vi "Main.vi"(8 "error in":errorcluster, 11 "TCP Listener in":refnum<class "DS TCP Listener.lvclass">) -> (0 "error out":errorcluster, 3 "TCP Listener out":refnum<class "DS TCP Listener.lvclass">)   [LabVIEW 2017, in "DS TCP Server.lvlib" / "DS TCP Listener.lvclass"]
doc: "The <b>Queued Message Handler</b> of the Worker that owns this VI."
uses:
  DS TCP Listener.lvclass
  Initialization Data.ctl
  Response Cases.ctl
  <vilib>/addons/_Workers/Library/Case Label.ctl
  DS TCP Listener.lvclass/DS TCP Listener.ctl
  rqp_Listen for Connections.ctl
  rsp_Add Listener.ctl
  rsp_New Connection.ctl
  <vilib>/addons/_Workers/Library/Classes/Message/Priority.ctl
  <vilib>/addons/_Workers/Library/Workers.lvlib
  <vilib>/addons/_Workers/Library/Classes/Message/Message.lvclass
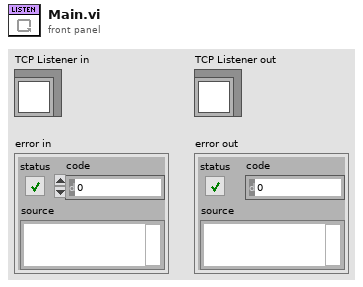
[diagram p1: front panel]
types:
  T1 = typedef "DS TCP Server.lvlib/DS TCP Listener.lvclass/Initialization Data.ctl" = cluster{"Response Cases":T2}
  T2 = typedef "DS TCP Server.lvlib/DS TCP Listener.lvclass/Response Cases.ctl" = cluster{"Add Listener":T3, "New Connection":T3}
  T3 = typedef "Workers.lvlib/Case Label.ctl" = string
  T4 = typedef "DS TCP Server.lvlib/DS TCP Listener.lvclass/rsp_Add Listener.ctl" = cluster{"listener ID":refnum<k5>, "Port":u16}
  T5 = typedef "DS TCP Server.lvlib/DS TCP Listener.lvclass/rqp_Listen for Connections.ctl" = cluster{"Server Name":string, "Port":u16}
  T6 = typedef "DS TCP Server.lvlib/DS TCP Listener.lvclass/rsp_New Connection.ctl" = cluster{"Connection Ref":refnum<k5>, "Name":string, "Message Priority":T7, "IP Address":string}
  T7 = typedef "Workers.lvlib/Message.lvclass/Priority.ctl" = enum16{"Low", "Normal", "High"}
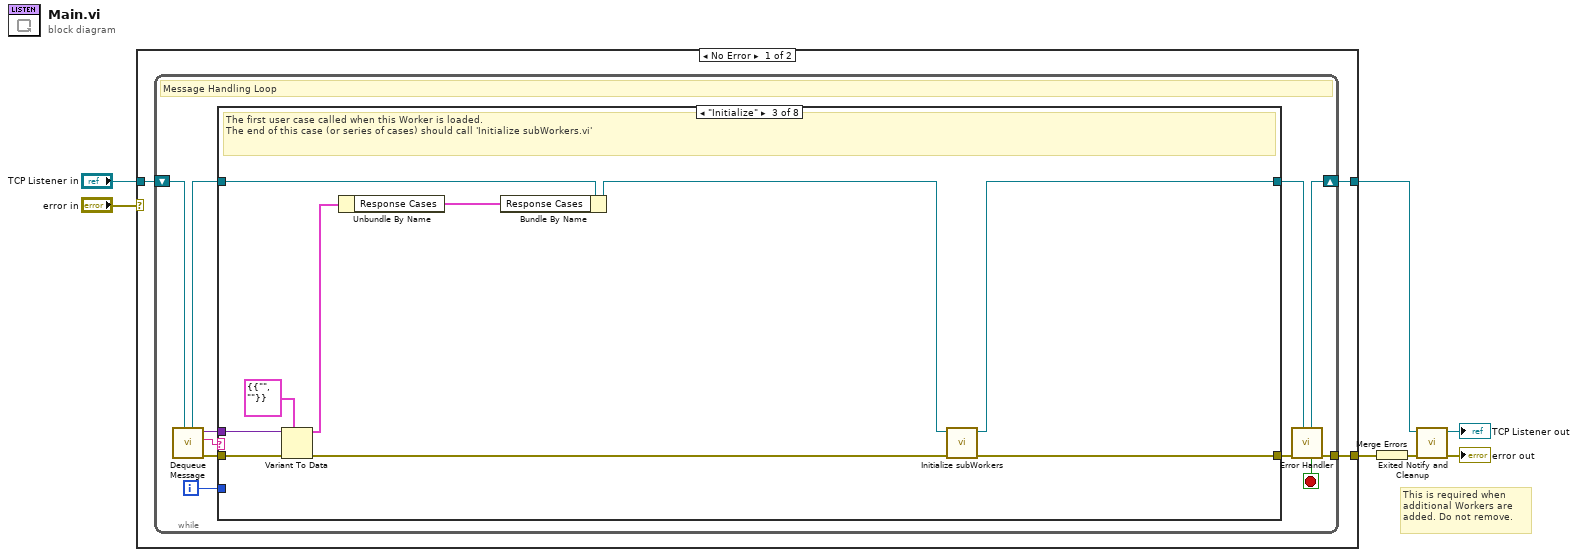
[diagram p0: block diagram]
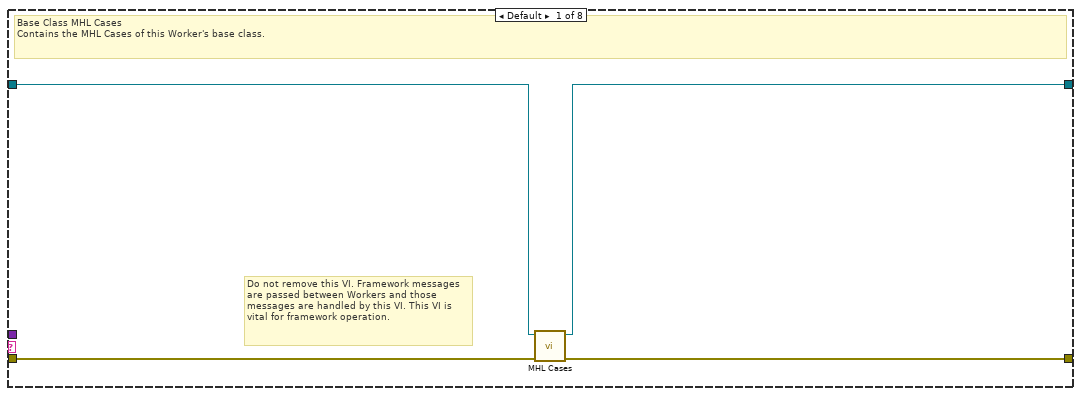
[diagram p2: hidden frame]
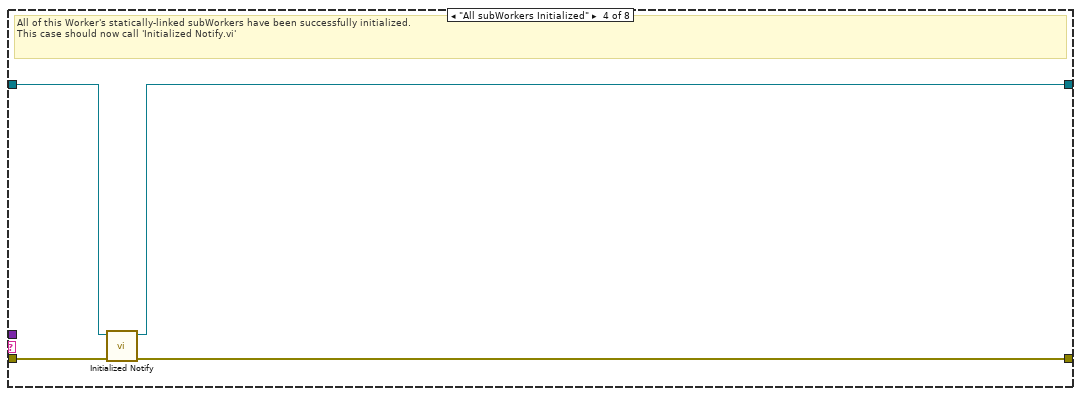
[diagram p4: hidden frame]
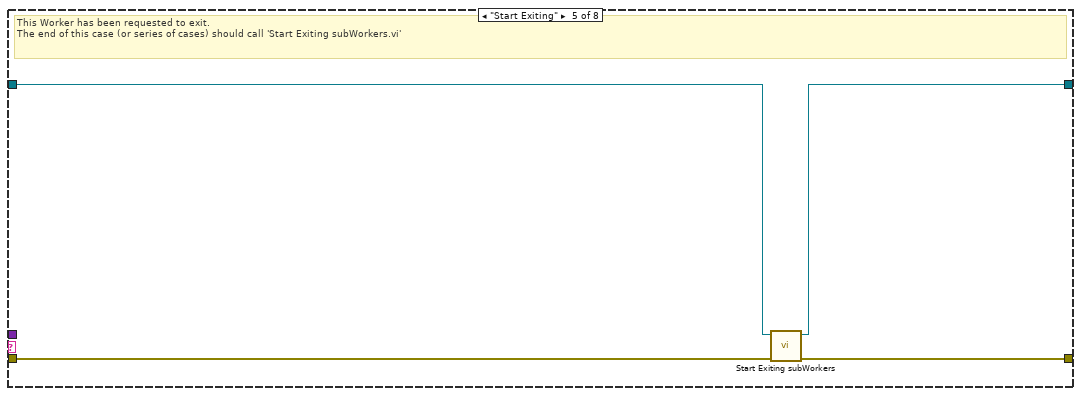
[diagram p5: hidden frame]
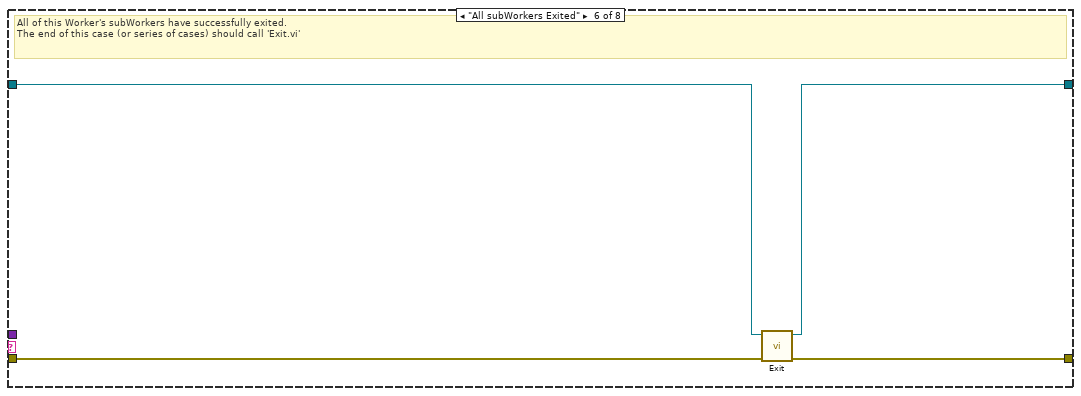
[diagram p6: hidden frame]
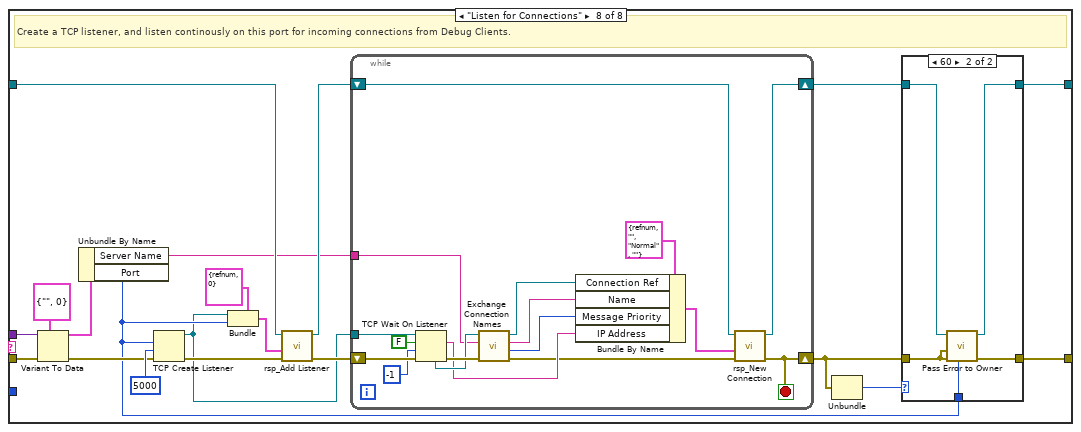
[diagram p8: hidden frame]
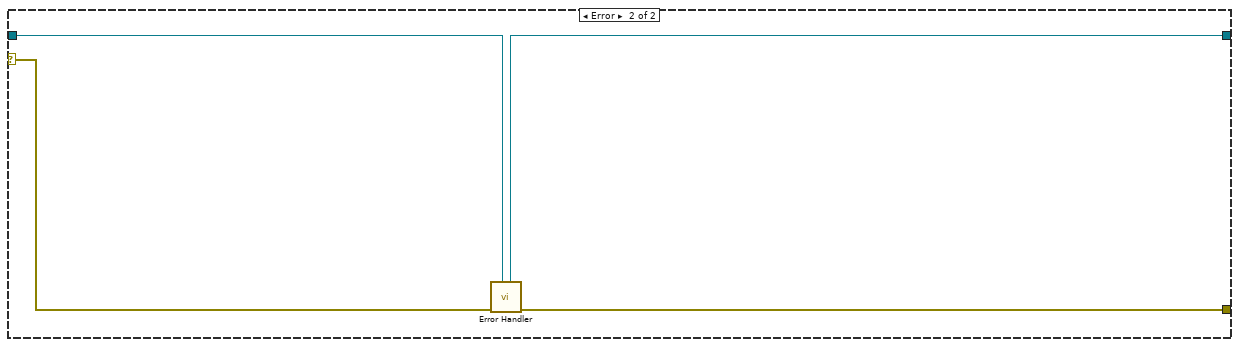
[diagram p10: hidden frame]
diagram:
  # "This is required when additional Workers are added. Do not remove."
  n1 = case shown="No Error" "error in" {
    tunnel: "TCP Listener in" -> [w8 w97]
    tunnel: [w10 w98] -> w6
    tunnel: [w9 w96] -> w7
    selector: "error in" -> [_ w99]
    frame No Error {
      n2 = while {
        shift-right: [w19] -> w9
        shift-left: w8 -> [w21]
        tunnel: [w20] -> w10
        i -> [w12]
        stop <- w13 stop-if-true
        # "Message Handling Loop"
        n3 = call-dynamic "Dequeue Message.vi"("Worker"=w21) -> ("error out"=w18:errorcluster, "Case out"=w14:string, "Data out"=w11:variant, "Worker out"=w16:refnum<class "DS TCP Listener.lvclass">)  [unwired: 6 in, 1 out]
        n4 = case "Worker MHL Case Structure (DO NOT CHANGE LABEL NAME)" shown="\"Initialize\"" w14 {
          tunnel: w18 -> [w25 w26 w35 w41 w42 w49 w51 w70]
          tunnel: [w24 w26 w37 w40 w45 w48 w51 w65] -> w17
          tunnel: w16 -> [w23 w27 w34 w39 w43 w47 w50 w62]
          tunnel: [w22 w27 w36 w38 w44 w46 w50 w68] -> w15
          tunnel: w12 -> [_ _ _ _ _ _ _ _]
          tunnel: w11 -> [_ _ w32 _ _ _ _ w59]
          frame Default {
            # "Do not remove this VI. Framework messages are passed between Workers and those messages are handled by this VI. This VI is vital for framework operation."
            # "Base Class MHL Cases\nContains the MHL Cases of this Worker's base class."
            n5 = call-dynamic "MHL Cases.vi"("error in"=w25, "Worker in"=w23) -> ("error out"=w24:errorcluster, "Worker out"=w22:refnum<class "DS TCP Listener.lvclass">)  [unwired: 8 in]
          }
          frame "------------ FRAMEWORK CASES -----------" {
            # "Start of Workers Framework Cases"
          }
          frame "Initialize" {
            # "The first user case called when this Worker is loaded.\nThe end of this case (or series of cases) should call 'Initialize subWorkers.vi'"
            n6 = Variant To Data(error in=w35, type=T1 {"Response Cases"={"Add Listener"="", "New Connection"=""}} ("Cluster"), Variant=w32) -> (data=w29:T1, error out=w33:errorcluster)
            n7 = Unbundle By Name(w29) -> ("Response Cases"=w28:T2)
            n8 = Bundle By Name(cluster=w34, "Response Cases"=w28) -> (w31:refnum<class "DS TCP Listener.lvclass">)
            n9 = call-dynamic "Initialize subWorkers.vi"("error in"=w33, "Worker"=w31) -> ("error out"=w37:errorcluster, "dup Worker out"=w36:refnum<class "DS TCP Listener.lvclass">)  [unwired: 8 in]
          }
          frame "All subWorkers Initialized" {
            # "All of this Worker's statically-linked subWorkers have been successfully initialized.\nThis case should now call 'Initialized Notify.vi'"
            n10 = call-dynamic "Initialized Notify.vi"("error in"=w41, "Worker"=w39) -> ("error out"=w40:errorcluster, "dup Worker out"=w38:refnum<class "DS TCP Listener.lvclass">)  [unwired: 8 in]
          }
          frame "Start Exiting" {
            # "This Worker has been requested to exit. \nThe end of this case (or series of cases) should call 'Start Exiting subWorkers.vi'"
            n11 = call-dynamic "Start Exiting subWorkers.vi"("error_in"=w42, "Worker"=w43) -> ("error out"=w45:errorcluster, "dup Worker out"=w44:refnum<class "DS TCP Listener.lvclass">)  [unwired: 8 in]
          }
          frame "All subWorkers Exited" {
            # "All of this Worker's subWorkers have successfully exited. \nThe end of this case (or series of cases) should call 'Exit.vi'"
            n12 = call-dynamic "Exit.vi"("error_in"=w49, "Worker"=w47) -> ("error out"=w48:errorcluster, "dup Worker out"=w46:refnum<class "DS TCP Listener.lvclass">)  [unwired: 8 in]
          }
          frame "------------- PUBLIC API CASES -------------" {
            # "Start of Public API Cases"
          }
          frame "Listen for Connections" {
            # "Create a TCP listener, and listen continously on this port for incoming connections from Debug Clients."
            n13 = Variant To Data(error in=w70, type=T5 {"Server Name"="", "Port"=0} ("Data"), Variant=w59) -> (data=w57:T5, error out=w60:errorcluster)
            n14 = Unbundle By Name(w57) -> ("Server Name"=w56:string, "Port"=w55:u16)
            n15 = TCP Create Listener(8:w60, 9:5000 ("timeout ms (25000)"), 10:w55) -> (0:w61:errorcluster, 3:w54:refnum<k5>)  [unwired: 3 out]
            n16 = Bundle(cluster=T4 {"listener ID"=refnum, "Port"=0} ("Cluster"), "listener ID"=w54, "Port"=w55) -> (w53:T4)
            n17 = call "rsp_Add Listener.vi"("error in"=w61, "Data in"=w53, "DS TCP Listener in"=w62) -> ("error out"=w64:errorcluster, "dup DS TCP Listener out"=w63:refnum<class "DS TCP Listener.lvclass">)  [unwired: 7 in]
            n18 = while {
              shift-right: [w83] -> w67
              shift-left: w63 -> [w82]
              shift-right: [w84] -> w66
              shift-left: w64 -> [w95]
              tunnel: w54 -> [w94]
              tunnel: w56 -> [w89]
              stop <- w84 stop-if-true
              n19 = TCP Wait On Listener(8:w95, 9:-1 ("timeout ms (wait forever: -1)"), 10:FALSE ("resolve remote address (T)"), 11:w94) -> (0:w91:errorcluster, 2:w86:string, 4:w90:refnum<k5>)  [unwired: 2 out]
              n20 = call "Exchange Connection Names.vi"("error in (no error)"=w91, "This Connection Name in"=w89, "connection ID"=w90) -> ("error out"=w81:errorcluster, "Message Priority"=w87:T7, "Remote Connection Name out"=w88:string, "connection out"=w92:refnum<k5>)  [unwired: 5 in]
              n21 = Bundle By Name(cluster=T6 {"Connection Ref"=refnum, "Name"="", "Message Priority"=enum."Normal", "IP Address"=""} ("Data"), "Connection Ref"=w92, "Name"=w88, "Message Priority"=w87, "IP Address"=w86) -> (w79:T6)
              n22 = call "rsp_New Connection.vi"("error in"=w81, "Data in"=w79, "DS TCP Listener in"=w82) -> ("error out"=w84:errorcluster, "dup DS TCP Listener out"=w83:refnum<class "DS TCP Listener.lvclass">)  [unwired: 7 in]
            }
            n23 = Unbundle(w66) -> ("code"=w69:i32)  [unwired: 2 out]
            n24 = case shown="60" w69 {
              tunnel: [w73 w76] -> w68
              tunnel: w67 -> [w73 w77]
              tunnel: w66 -> [w72 w75]
              tunnel: [w72 w78] -> w65
              tunnel: w55 -> [_ w74]
              frame Default {
              }
              frame 60 {
                n25 = call-dynamic "Pass Error to Owner.vi"("Auxiliary"=w74, "error_in"=w75, "Error to Pass to Owner"=w75, "Worker"=w77) -> ("error out"=w78:errorcluster, "dup Worker out"=w76:refnum<class "DS TCP Listener.lvclass">)  [unwired: 6 in]
              }
            }
          }
        }
        n26 = call-dynamic "Error Handler.vi"("Worker"=w15, "error_in"=w17) -> ("error out"=w20:errorcluster, "Stop Loop"=w13:bool, "Worker out"=w19:refnum<class "DS TCP Listener.lvclass">)  [unwired: 7 in]
      }
    }
    frame Error {
      n27 = call-dynamic "Error Handler.vi"("Worker"=w97, "error_in"=w99) -> ("error out"=w98:errorcluster, "Worker out"=w96:refnum<class "DS TCP Listener.lvclass">)  [unwired: 7 in, 1 out]
    }
  }
  n28 = Merge Errors(w6) -> (w3:errorcluster)
  n29 = call-dynamic "Exited Notify and Cleanup.vi"("error_in"=w3, "Worker"=w7) -> ("error out"=→"error out":errorcluster, "dup Worker out"=→"TCP Listener out":refnum<class "DS TCP Listener.lvclass">)  [unwired: 8 in]
